vi "SubVI_HELP.vi"() -> ()   [LabVIEW 2014]
panel:
  in  "1 10":u32(colorbox)=16777215
  in  "1 9":u32(colorbox)=8421504
  in  "1 8":u32(colorbox)=8323199
  in  "1 7":u32(colorbox)=255
  in  "1 6":u32(colorbox)=65280
  in  "1 5":u32(colorbox)=16776960
  in  "1 4":u32(colorbox)=16744192
  in  "1 3":u32(colorbox)=16711680
  in  "1 2":u32(colorbox)=10824192
  in  "1":u32(colorbox)
  in  "Enter":bool
  # "堵"
  # "茨"
  # "¬õ"
  # "卷"
  # "独"
  # "厚"
  # "屡"
  # "档"
  # "η"
  # "フ"
  # "¹qªýÃC¦â"
  # "0"
  # "1"
  # "2"
  # "3"
  # "4"
  # "5"
  # "6"
  # "7"
  # "8"
  # "9"
  # "¹ïÀ³¼Æ¦r"
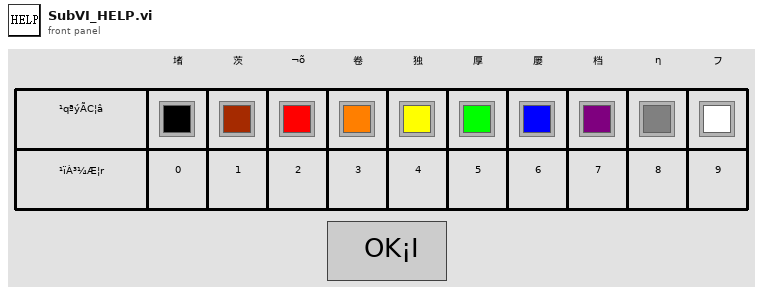
[diagram p1: front panel]
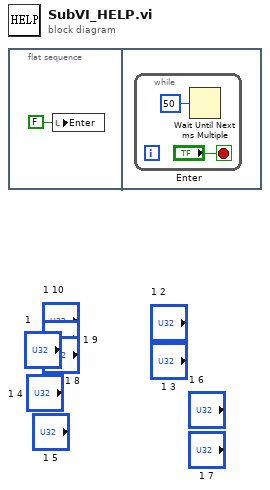
[diagram p0: block diagram]
diagram:
  n1 = flat-sequence {
    frame #0 {
      n2 = local write "Enter"(FALSE ("Enter")) -> ()
    }
    frame #1 {
      n3 = while {
        stop <- "Enter" stop-if-true
        n4 = Wait Until Next ms Multiple(millisecond multiple=u32 50 ("milliseconds to wait")) -> ()  [unwired: 1 out]
      }
    }
  }
